vi "BPF Spectrum.vi"(8 "error in (no error)":errorcluster, 9 "Depth":u32=50, 10 "Window Width":u32=10, 11 "Spectral Processing in":refnum<class "Spectral Processing.lvclass">) -> (0 "error out":errorcluster, 3 "Spectral Processing out":refnum<class "Spectral Processing.lvclass">)   [LabVIEW 2014, in "Spectral Processing.lvclass"]
uses:
  Spectral Processing.lvclass
  <vilib>/Analysis/3filter.llb/Filter Passband Type.ctl
  Spectral Processing.lvclass/Spectral Processing.ctl
  <vilib>/Analysis/4window.llb/Hanning Window (DBL).vi
  <vilib>/Analysis/baseanly.llb/Quick Scale 1D.vi
  <vilib>/Analysis/2dsp.llb/Inverse Real FFT.vi
  <vilib>/Analysis/4window.llb/AllCosWindow (DBL).vi
  <vilib>/Analysis/3filter.llb/IIR Filter (DBL).vi
  <vilib>/Analysis/3filter.llb/Butterworth Filter (DBL).vi
  <vilib>/Analysis/3filter.llb/Zero Phase Filter (DBL).vi
  <vilib>/Analysis/NI_AALPro.lvlib
  <vilib>/Analysis/NI_AALBase.lvlib
panel:
  out "Processed Spectrum":dbl[][](graph)
  out "Fourier Domain":dbl[][](graph)
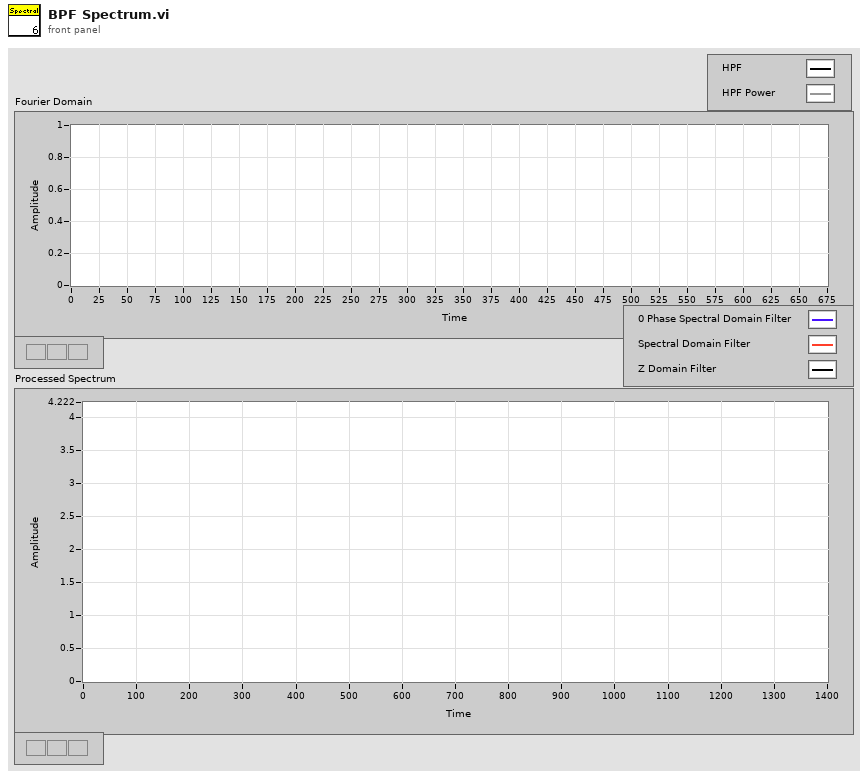
[diagram p1: front panel]
types:
  T1 = typedef "NI_AALBase.lvlib/Filter Passband Type.ctl" = enum32{"Lowpass", "Highpass", "Bandpass", "Bandstop"}
  T2 = cluster{"filter structure":enum32{"IIR 2nd Order", "IIR 4th Order"}, "Reverse Coefficients":dbl[], "Forward Coefficients":dbl[]}
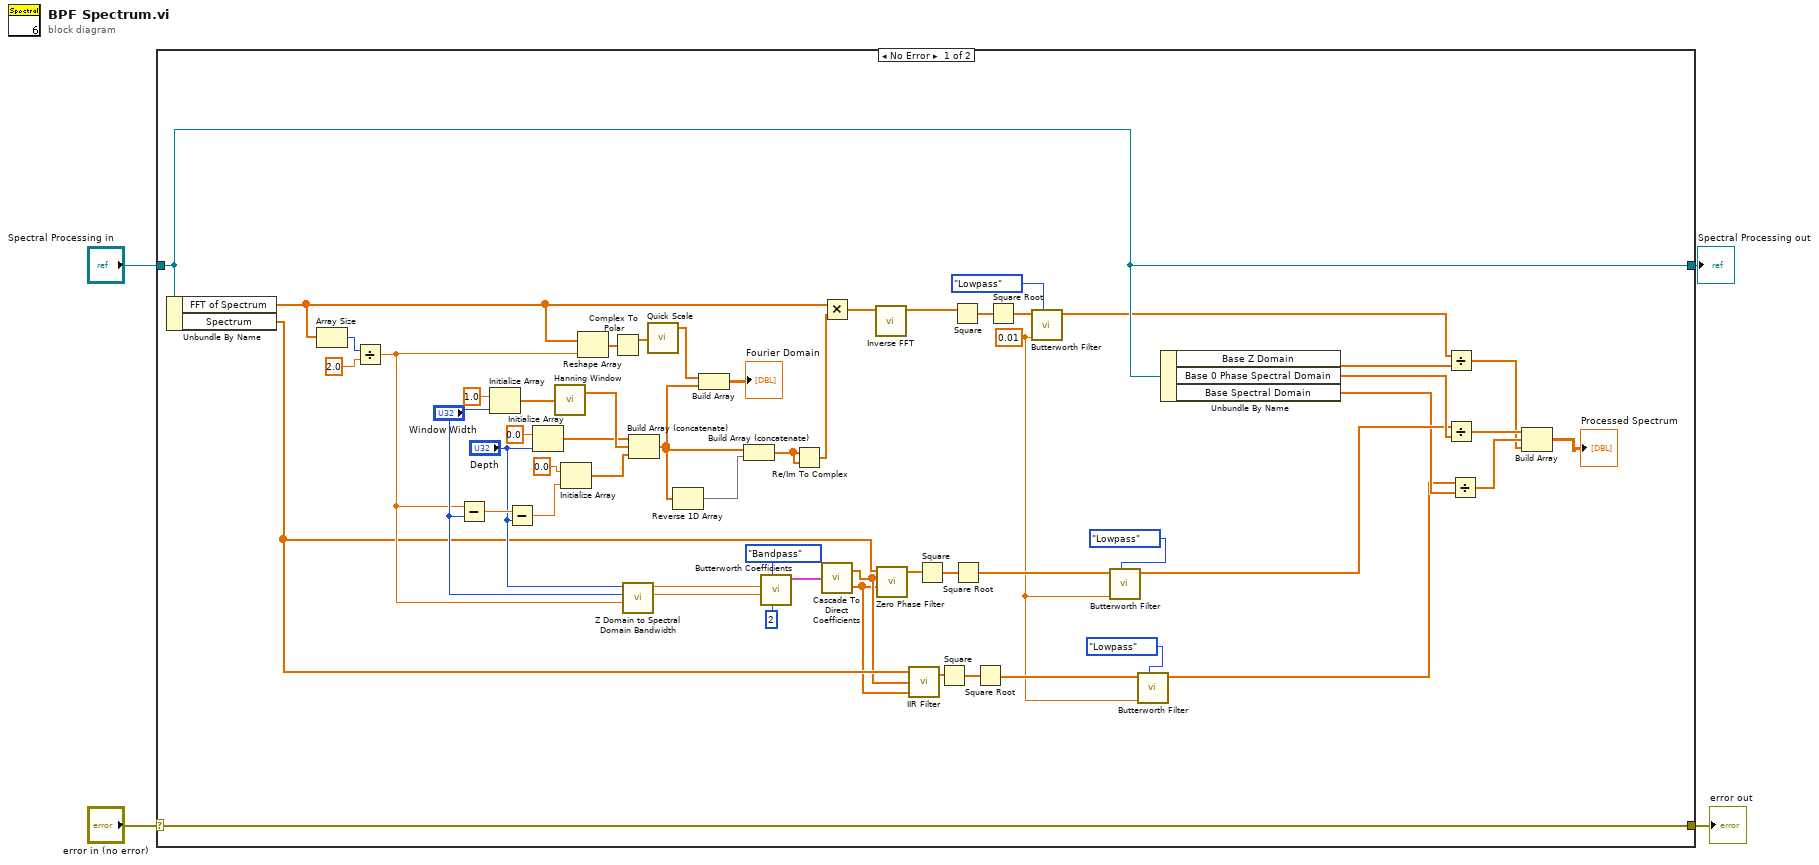
[diagram p0: block diagram]
diagram:
  n1 = case shown="No Error" "error in (no error)" {
    selector: "error in (no error)" -> [w61 w63]
    tunnel: [w61 w63] -> w3
    tunnel: [w15 w62] -> w1
    tunnel: "Spectral Processing in" -> [w15 w62]
    frame No Error {
      w19 = 0.01 ("low cutoff freq: fl")
      n2 = Unbundle By Name(w15) -> ("FFT of Spectrum"=w48:cdb[], "Spectrum"=w29:dbl[])
      n3 = Array Size(array=w48) -> (size(s)=w35:i32)
      n4 = Divide(x=w35, y=2.0 ("element")) -> (x/y=w31:dbl)
      n5 = Subtract(x=w31, y="Window Width") -> (x-y=w56:dbl)
      n6 = Initialize Array(1.0 ("element"), "Window Width") -> (w60:dbl[])
      n7 = Subtract(x=w56, y="Depth") -> (x-y=w55:dbl)
      n8 = Initialize Array(0.0 ("element"), "Depth") -> (w53:dbl[])
      n9 = call-poly <vilib>:"Hanning Window.vi"("X"=w60) -> ("Windowed X"=w54:dbl[])  [unwired: 1 out]
      n10 = Initialize Array(0.0 ("element"), w55) -> (w52:dbl[])
      n11 = Reshape Array(w48, w31) -> (w47:cdb[])
      n12 = Complex To Polar(r * e^(i*theta)=w47) -> (r=w46:dbl[])  [unwired: 1 out]
      n13 = call "Z Domain to Spectral Domain Bandwidth.vi"("Samples"=w31, "Window Width"="Window Width", "Depth"="Depth") -> ("Low Pass Freq (scaled)"=w32:dbl, "High Pass Freq (Scaled)"=w33:dbl)  [unwired: 7 in]
      n14 = Build Array (concatenate)(w53, w54, w52) -> (w49:dbl[])
      n15 = call-poly <vilib>:"Quick Scale.vi"("X"=w46) -> ("Y[i]=X[i]/Max|X|"=w45:dbl[])  [unwired: 2 out]
      n16 = Reverse 1D Array(array=w49) -> (reversed array=w50:dbl[])
      n17 = Build Array(w45, w49) -> (→"Fourier Domain":dbl[][])
      n18 = Build Array (concatenate)(w49, w50) -> (w30:dbl[])
      n19 = call <vilib>:"Butterworth Coefficients.vi"("order"=2, "filter type"=Filter_Passband_Type."Bandpass", "low cutoff freq: fl"=w32, "high cutoff freq: fh"=w33) -> ("IIR Filter Cluster"=w44:T2)  [unwired: 6 in, 1 out]
      n20 = Re/Im To Complex(1:w30, 2:w30) -> (0:w18:cdb[])
      n21 = Multiply(x=w48, y=w18) -> (x*y=w17:cdb[])
      n22 = call <vilib>:"Cascade To Direct Coefficients.vi"("IIR Filter Cluster"=w44) -> ("Reverse Coefficients"=w27:dbl[], "Forward Coefficients"=w26:dbl[])
      n23 = call-poly <vilib>:"Inverse FFT.vi"("FFT {X}"=w17) -> ("X"=w38:dbl[])  [unwired: 9 in, 1 out]
      n24 = call-poly <vilib>:"Zero Phase Filter.vi"("Forward Coefficients"=w26, "Reverse Coefficients"=w27, "X"=w29) -> ("Filtered X"=w41:dbl[])  [unwired: 7 in, 1 out]
      n25 = call-poly <vilib>:"IIR Filter.vi"("Forward Coefficients"=w26, "Reverse Coefficients"=w27, "X"=w29) -> ("Filtered X"=w28:dbl[])  [unwired: 1 in, 1 out]
      n26 = Square(x=w41) -> (x^2=w40:dbl[])
      n27 = Square(x=w28) -> (x^2=w34:dbl[])
      n28 = Square(x=w38) -> (x^2=w39:dbl[])
      n29 = Square Root(x=w40) -> (sqrt(x)=w24:dbl[])
      n30 = Square Root(x=w34) -> (sqrt(x)=w25:dbl[])
      n31 = Square Root(x=w39) -> (sqrt(x)=w23:dbl[])
      n32 = call-poly <vilib>:"Butterworth Filter.vi"("filter type"=Filter_Passband_Type."Lowpass", "low cutoff freq: fl"=w19, "X"=w23) -> ("Filtered X"=w6:dbl[])  [unwired: 5 in, 1 out]
      n33 = call-poly <vilib>:"Butterworth Filter.vi"("filter type"=Filter_Passband_Type."Lowpass", "low cutoff freq: fl"=w19, "X"=w24) -> ("Filtered X"=w13:dbl[])  [unwired: 5 in, 1 out]
      n34 = call-poly <vilib>:"Butterworth Filter.vi"("filter type"=Filter_Passband_Type."Lowpass", "low cutoff freq: fl"=w19, "X"=w25) -> ("Filtered X"=w11:dbl[])  [unwired: 5 in, 1 out]
      n35 = Unbundle By Name(w15) -> ("Base Z Domain"=w7:dbl[], "Base 0 Phase Spectral Domain"=w14:dbl[], "Base Spectral Domain"=w12:dbl[])
      n36 = Divide(x=w6, y=w7) -> (x/y=w8:dbl[])
      n37 = Divide(x=w13, y=w14) -> (x/y=w10:dbl[])
      n38 = Divide(x=w11, y=w12) -> (x/y=w9:dbl[])
      n39 = Build Array(w10, w9, w8) -> (→"Processed Spectrum":dbl[][])
    }
    frame Error {
    }
  }
  "error out" <- w3
  "Spectral Processing out" <- w1
